vi "Global Stop.vi"(7 "Command":T2=enum."Read", 8 "error in (no error)":errorcluster, 9 "Stop on Error?":bool=TRUE, 10 "Stop?":bool, 11 "Stop Ref":T1) -> (0 "error out":errorcluster, 2 "Latched Stop":bool, 3 "Stop Ref out":T1)   [LabVIEW 2013, in "J1939 Addon Engine.lvlib" / "Stop FG.lvlib"]
uses:
  Stop FG.lvlib
  Stop Global Commands.ctl
  Stop Global Ref.ctl
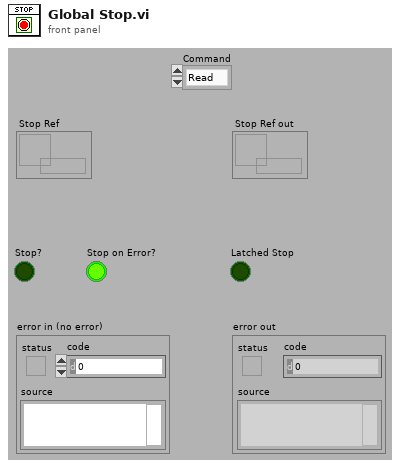
[diagram p1: front panel]
types:
  T1 = typedef "J1939 Addon Engine.lvlib/Stop FG.lvlib/Stop Global Ref.ctl" = refnum<data-value>
  T2 = typedef "J1939 Addon Engine.lvlib/Stop FG.lvlib/Stop Global Commands.ctl" = enum16{"Write", "Read", "Reset"}
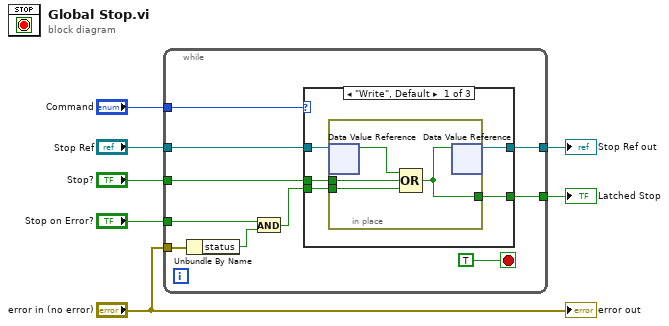
[diagram p0: block diagram]
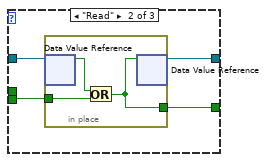
[diagram p2: hidden frame]
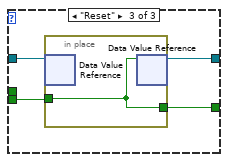
[diagram p3: hidden frame]
diagram:
  n1 = while {
    tunnel: "Stop?" -> [w16]
    tunnel: "Command" -> [w15]
    tunnel: "error in (no error)" -> [w14]
    tunnel: "Stop on Error?" -> [w12]
    tunnel: "Stop Ref" -> [w11]
    tunnel: [w9] -> w2
    tunnel: [w8] -> w1
    stop <- TRUE stop-if-true
    n2 = Unbundle By Name(w14) -> ("status"=w13:bool)
    n3 = And(x=w12, y=w13) -> (x .and. y?=w10:bool)
    n4 = case shown="\"Write\", Default" w15 {
      tunnel: [w21 w29 w37] -> w9
      tunnel: w16 -> [w22 _ _]
      tunnel: w11 -> [w20 w30 w35]
      tunnel: w10 -> [w19 w28 w36]
      tunnel: [w18 w27 w34] -> w8
      frame "Write", Default {
        n5 = in-place {
          in-place-border: w22 -> [w26]
          in-place-border: [w24] -> w21
          in-place-border: w19 -> [w23]
          n6 = in-place-dvr #1(w20) -> (w25:bool)  [unwired: 1 out]
          n7 = Compound Arithmetic op=OR(w25, w26, w23) -> (w24:bool)
          n8 = in-place-dvr #1(w24) -> (w18:T1)  [unwired: 1 out]
        }
      }
      frame "Read" {
        n9 = in-place {
          in-place-border: [w31] -> w29
          in-place-border: w28 -> [w32]
          n10 = in-place-dvr #2(w30) -> (w33:bool)  [unwired: 1 out]
          n11 = Or(x=w33, y=w32) -> (x .or. y?=w31:bool)
          n12 = in-place-dvr #2(w31) -> (w27:T1)  [unwired: 1 out]
        }
      }
      frame "Reset" {
        n13 = in-place {
          in-place-border: [w38] -> w37
          in-place-border: w36 -> [w38]
          n14 = in-place-dvr #3(w35) -> ()  [unwired: 2 out]
          n15 = in-place-dvr #3(w38) -> (w34:T1)  [unwired: 1 out]
        }
      }
    }
  }
  "Latched Stop" <- w2
  "Stop Ref out" <- w1
  "error out" <- "error in (no error)"
